vi "accumet data parser.vi"(8 "error in (no error)":errorcluster, 11 "Read String":string="SPL# 00001    00:02:09        TIC =  116.355  mV    000000  ug C    000000  ppm    \r\nSPL# 00001    00:02:12        TOC = 47.6076  mV    000000  ug C    000000  ppm \n") -> (0 "error out":errorcluster, 2 "numeric output":dbl[](array[numeric]), 3 "parsed ouput":string[](array[string]))   [LabVIEW 2010]
panel:
  in  "delimiter":string=" "
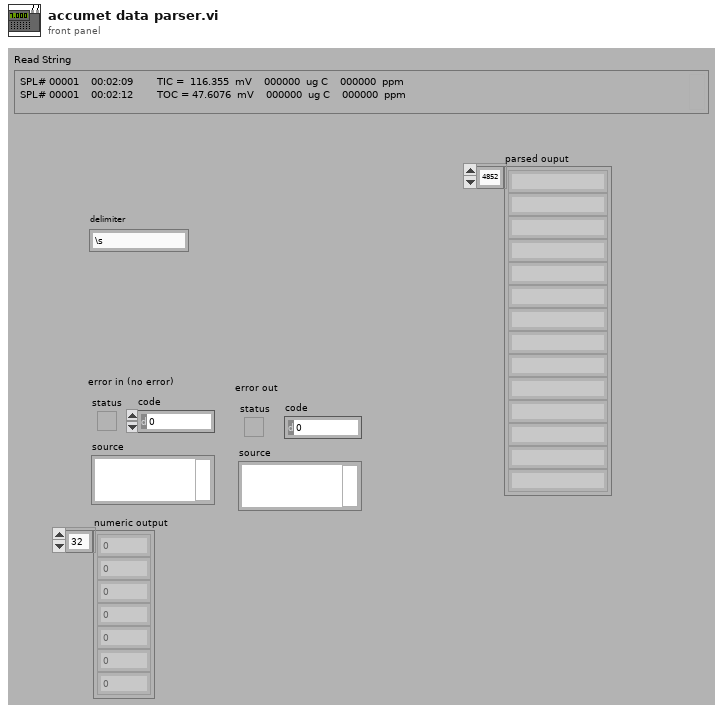
[diagram p1: front panel]
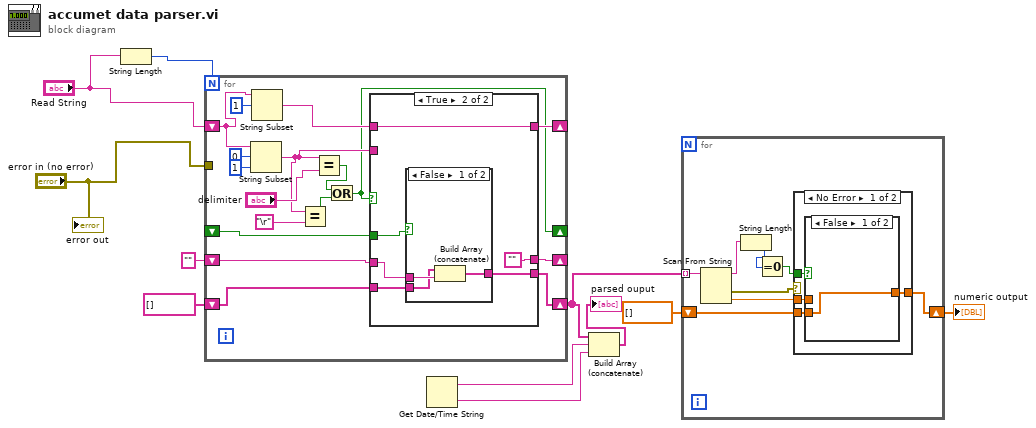
[diagram p0: block diagram]
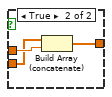
[diagram p2: hidden frame]
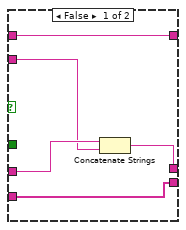
[diagram p4: hidden frame]
diagram:
  n1 = String Length(string="Read String") -> (length=w10:i32)
  n2 = for {
    N: w10 -> [_]
    tunnel: "error in (no error)" -> [_]
    shift-right: [w26] -> _
    shift-left: "Read String" -> [w23]
    shift-right: [w21] -> _
    shift-left: "" -> [w20]
    shift-right: [w16] -> _
    shift-left: _ -> [w14]
    shift-right: [w12] -> w6
    shift-left: string[] [] -> [w13]
    n3 = String Subset(string=w23, offset (0)=0, length (rest)=1 ("length (rest)")) -> (substring=w18:string)
    n4 = String Subset(string=w23, offset (0)=1) -> (substring=w22:string)  [unwired: 1 in]
    n5 = Equal?(x=w18, y="\r") -> (x = y?=w19:bool)
    n6 = Equal?(x=w18, y="delimiter") -> (x = y?=w15:bool)
    n7 = Or(x=w15, y=w19) -> (x .or. y?=w16:bool)
    n8 = case shown="True" w16 {
      tunnel: [w30 w39] -> w26
      tunnel: w22 -> [w30 w39]
      tunnel: [w33 ""] -> w21
      tunnel: w20 -> [w32 w36]
      tunnel: w18 -> [w31 _]
      tunnel: w14 -> [_ w37]
      tunnel: w13 -> [w29 w35]
      tunnel: [w29 w34] -> w12
      frame False {
        n9 = Concatenate Strings(w32, w31) -> (w33:string)
      }
      frame True {
        n10 = case shown="False" w37 {
          tunnel: w36 -> [w42 _]
          tunnel: w35 -> [w41 w43]
          tunnel: [w40 w43] -> w34
          frame False {
            n11 = Build Array (concatenate)(w41, w42) -> (w40:string[])
          }
          frame True {
          }
        }
      }
    }
  }
  n12 = Get Date/Time String() -> (date string=w8:string, time string=w7:string)  [unwired: 3 in]
  n13 = Build Array (concatenate)(w6, w8, w7) -> (→"parsed ouput":string[])
  n14 = for {
    tunnel: w6 -> [w51] mode=indexing
    shift-right: [w48] -> w9
    shift-left: dbl[] [] -> [w47]
    n15 = Scan From String(input string=w51) -> (remaining string=w46:string, error out=w50:errorcluster, output 1=w49:dbl)  [unwired: 4 in, 1 out]
    n16 = String Length(string=w46) -> (length=w45:i32)
    n17 = Equal To 0?(x=w45) -> (x = 0?=w44:bool)
    n18 = case shown="No Error" w50 {
      tunnel: w49 -> [w55 _]
      tunnel: [w54 w60] -> w48
      tunnel: w47 -> [w53 w60]
      tunnel: w44 -> [w52 _]
      frame No Error {
        n19 = case shown="False" w52 {
          tunnel: w55 -> [_ w59]
          tunnel: [w56 w58] -> w54
          tunnel: w53 -> [w56 w57]
          frame False {
          }
          frame True {
            n20 = Build Array (concatenate)(w57, w59) -> (w58:dbl[])
          }
        }
      }
      frame Error {
      }
    }
  }
  "numeric output" <- w9
  "error out" <- "error in (no error)"
